vi "m100ProgramCheck.vi"() -> ()   [LabVIEW 2012]
uses:
  <vilib>/addons/database/Auxilliary.llb/DB Tools Cursor Type.ctl
  <vilib>/addons/database/Connection.llb/DB Tools Open Connec (Path).vi
  <vilib>/addons/database/Connection.llb/Conn Execute.vi
  <vilib>/addons/database/Recordset.llb/Rec Fetch Recordset Data (R).vi
  <vilib>/addons/database/Recordset.llb/Rec Destroy - Connection.vi
  <vilib>/addons/database/Recordset.llb/Rec Fetch String Data (R).vi
  <vilib>/addons/database/Recordset.llb/Rec Fetch Integer Data (R).vi
  <vilib>/addons/database/_DB Variant To Data/Database Variant To Data.xnode
  <vilib>/addons/database/NI_Database_API.lvlib
  <vilib>/Utility/SMTP/NI_SMTPEmail.lvlib
panel:
  out "x = y?":bool
  out "data":i32
  out "array":string[][](array[string])
  out "concatenated string 2":string
  out "concatenated string":string
  out "data 5":string
  out "error out":errorcluster
  out "recordset data":variant[][](array[variant])
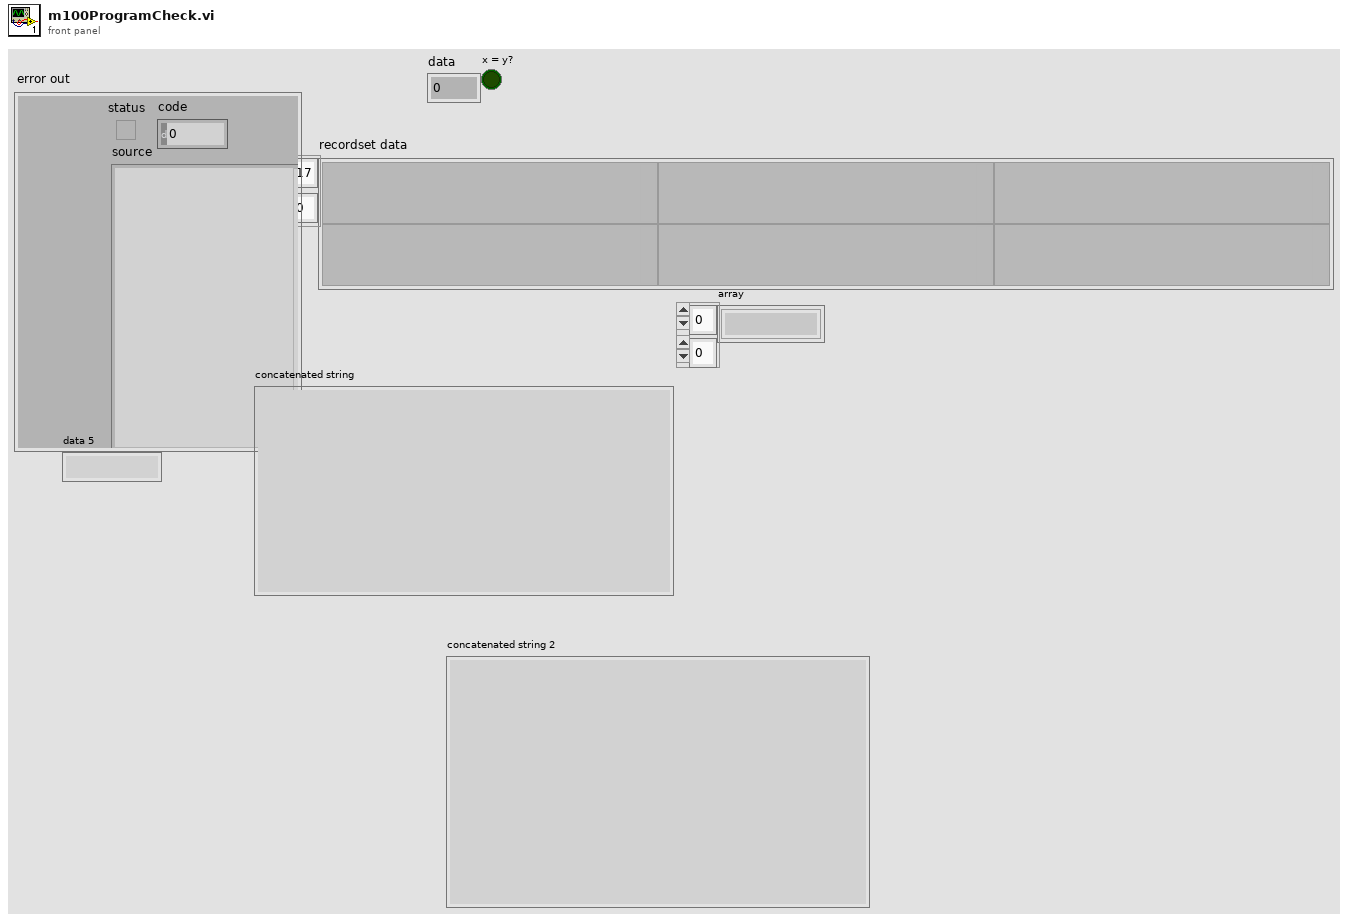
[diagram p1: front panel]
types:
  T1 = typedef "NI_Database_API.lvlib/DB Tools Cursor Type.ctl" = enum16{"forward-only", "keyset", "dynamic", "static"}
  T2 = typedef "NI_Database_API.lvlib/Conn ObjectReference.ctl" = refnum<k1>
  T3 = typedef "NI_Database_API.lvlib/Rec ObjectReference.ctl" = refnum<k1>
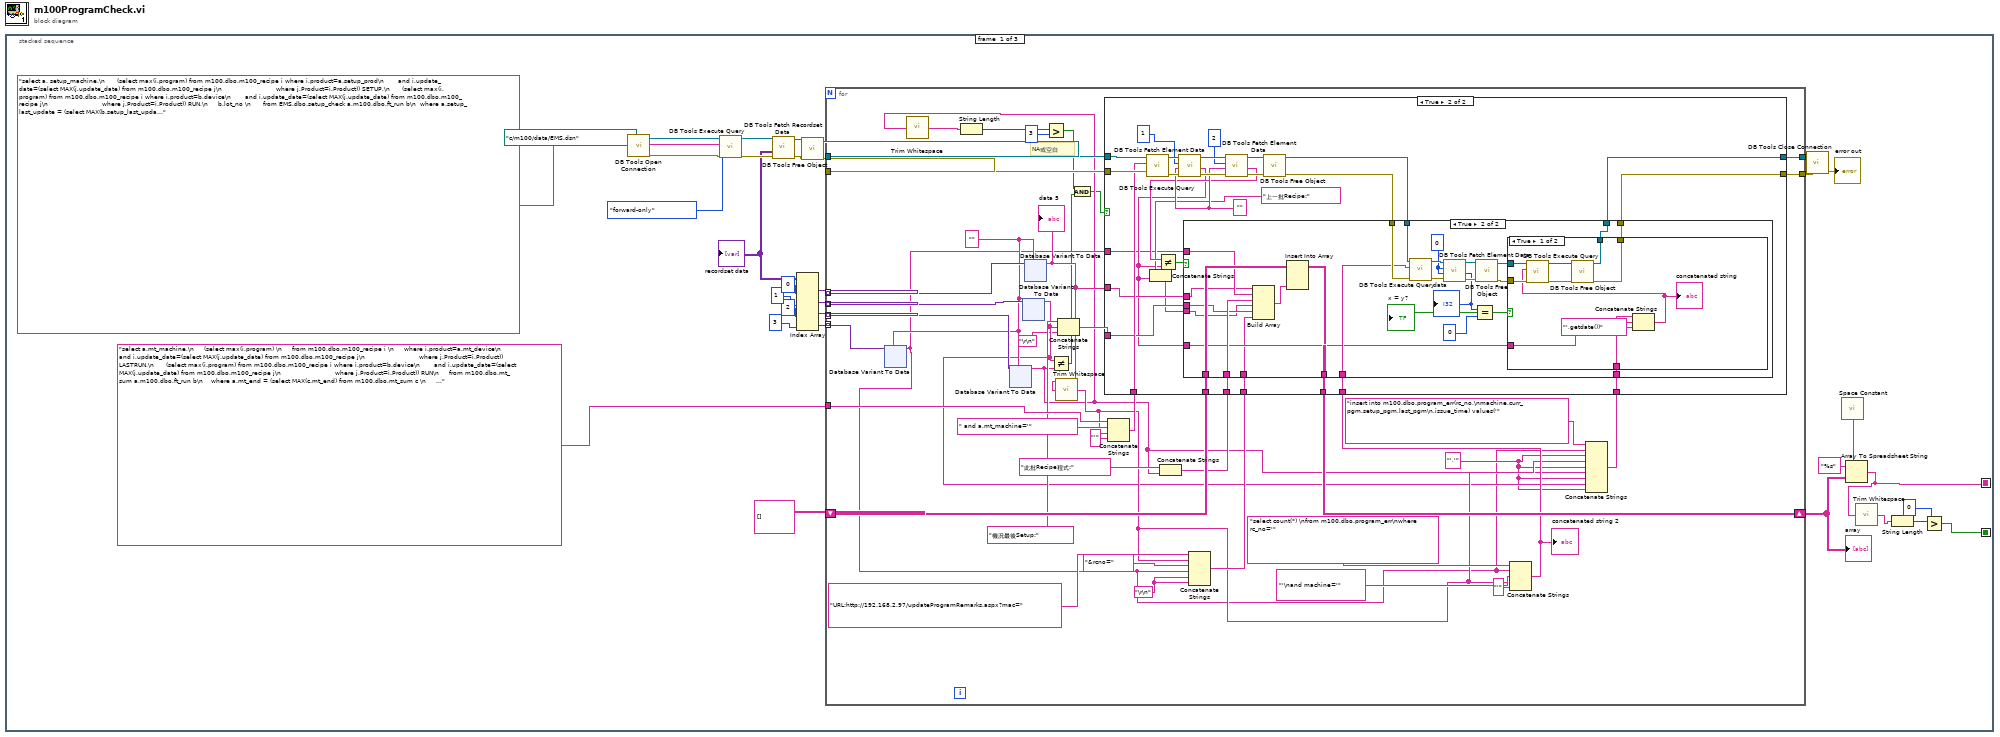
[diagram p0: block diagram]
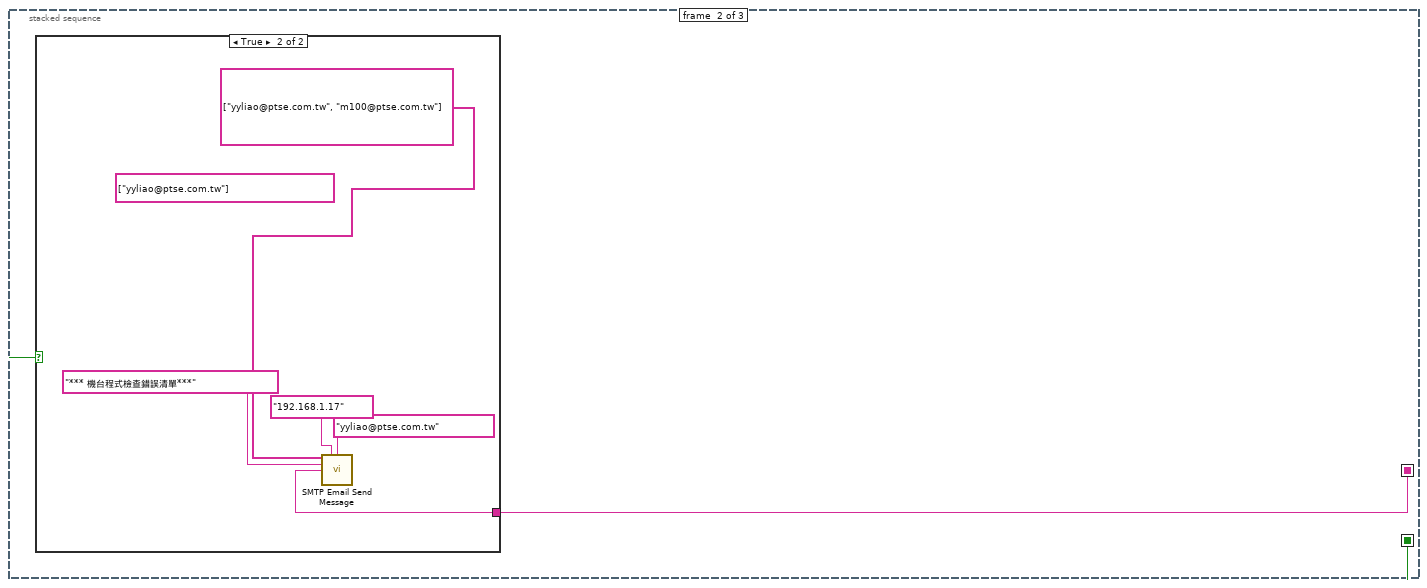
[diagram p5: hidden frame]
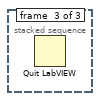
[diagram p7: hidden frame]
diagram:
  n1 = stacked-sequence {
    seq-local: [w5 _ _] -> [_ w279 _]
    seq-local: [w1 _ _] -> [_ w278 _]
    frame #0 {
      n2 = call-poly <vilib>:"DB Tools Open Connection.vi"("connection information"=path "c:/m100/data/EMS.dsn") -> ("error out"=w12:errorcluster, "connection reference"=w13:T2)  [unwired: 7 in]
      n3 = call-poly <vilib>:"DB Tools Execute Query.vi"("error in (no error)"=w12, "cursor type"=DB_Tools_Cursor_Type."forward-only", "SQL query"="select a. setup_machine,\n      (select max(i.program) from m100.dbo.m100_recipe i where i.product=a.setup_prod\n       and i.update_date=(select MAX(j.update_date) from m100.dbo.m100_recipe j\n                           where j.Product=i.Product)) SETUP,\n      (select max(i.program) from m100.dbo.m100_recipe i where i.product=b.device\n       and i.update_date=(select MAX(j.update_date) from m100.dbo.m100_recipe j\n                           where j.Product=i.Product)) RUN,\n     b.lot_no \n      from EMS.dbo.setup_check a,m100.dbo.ft_run b\n  where a.setup_last_update = (select MAX(b.setup_last_update) from EMS.dbo.setup_check b\n                               where b.setup_machine=a.setup_machine)\n    and a.setup_machine=b.machine\n    and b.lot_no like 'A%'\n    and b.station='MT'\n    and b.lot_no not in (select d.rc_no from m100.dbo.program_err d \n                         where d.machine = b.machine\n                           and LEN(d.owner) > 0)\norder by a.setup_machine", "connection reference"=w13) -> ("error out"=w31:errorcluster, "recordset reference"=w32:T3)  [unwired: 4 in]
      n4 = call-poly <vilib>:"DB Tools Fetch Recordset Data.vi"("error in (no error)"=w31, "recordset reference"=w32) -> ("error out"=w29:errorcluster, "recordset data"=w26:variant[][], "recordset reference out"=w30:T3)  [unwired: 3 in]
      "recordset data" <- w26
      n5 = Index Array(array=w26, index (col) #1=0 ("disabled index (col)"), index (col) #2=1 ("index (col)"), index (col) #3=2 ("index (col)"), index (col) #4=3 ("index (col)")) -> (element #1=w22:variant[], element #2=w21:variant[], element #3=w20:variant[], element #4=w6:variant[])  [unwired: 4 in]
      n6 = call-poly <vilib>:"DB Tools Free Object.vi"("error in (no error)"=w29, "recordset reference"=w30) -> ("error out"=w16:errorcluster, "connection reference"=w17:T2)  [unwired: 8 in]
      n7 = for {
        tunnel: w22 -> [w75] mode=indexing
        tunnel: w21 -> [w74] mode=indexing
        tunnel: w20 -> [w73] mode=indexing
        shift-right: [w62] -> w8
        shift-left: string[][] [] ("array") -> [w65]
        tunnel: w17 -> [w72]
        tunnel: w16 -> [w71]
        tunnel: [w70] -> w15
        tunnel: [w69] -> w14
        tunnel: "select a.mt_machine,\n     (select max(i.program) \n     from m100.dbo.m100_recipe i \n     where i.product=a.mt_device\n       and i.update_date=(select MAX(j.update_date) from m100.dbo.m100_recipe j\n                           where j.Product=i.Product)) LASTRUN,\n      (select max(i.program) from m100.dbo.m100_recipe i where i.product=b.device\n       and i.update_date=(select MAX(j.update_date) from m100.dbo.m100_recipe j\n                           where j.Product=i.Product)) RUN\n     from m100.dbo.mt_sum a,m100.dbo.ft_run b\n    where a.mt_end = (select MAX(c.mt_end) from m100.dbo.mt_sum c \n                       where c.mt_machine=a.mt_machine)\n      and a.mt_machine=b.machine\n      and b.station='MT'     " -> [w68]
        tunnel: w6 -> [w56] mode=indexing
        w41 = "\r\n"
        w44 = "','" ("string")
        w55 = ""
        # "NA或空白"
        n8 = xnode "Database Variant To Data"("database variant"=w56, "type"=w55) -> ("data"=w43:string)  [unwired: 1 in, 1 out]
        n9 = xnode "Database Variant To Data"("database variant"=w73, "type"=w55) -> ("data"=w40:string)  [unwired: 1 in, 1 out]
        n10 = call <vilib>:"Trim Whitespace.vi"("string"=w40) -> ("trimmed string"=w39:string)  [unwired: 1 in]
        n11 = String Length(string=w39) -> (length=w38:i32)
        n12 = xnode "Database Variant To Data"("database variant"=w74, "type"=w55) -> ("data"=w46:string)  [unwired: 1 in, 1 out]
        n13 = xnode "Database Variant To Data"("database variant"=w75, "type"=w55) -> ("data"=w63:string)  [unwired: 1 in, 1 out]
        "data 5" <- w63
        n14 = Greater?(x=w38, y=3) -> (0:w36:bool)
        n15 = Not Equal?(x=w46, y=w40) -> (x != y?=w35:bool)
        n16 = call <vilib>:"Trim Whitespace.vi"("string"=w63) -> ("trimmed string"=w47:string)  [unwired: 1 in]
        n17 = Concatenate Strings("機況最後Setup:" ("string"), w46, "\r\n") -> (w58:string)
        n18 = And(x=w36, y=w35) -> (x .and. y?=w34:bool)
        n19 = Concatenate Strings(w68, " and a.mt_machine='" ("string"), w47, "'" ("string")) -> (w66:string)
        n20 = Concatenate Strings("此批Recipe程式:" ("string"), w40) -> (w60:string)
        n21 = Concatenate Strings("URL:http://192.168.2.97/updateProgramRemarks.aspx?mac=" ("string"), w47, "&rcno=" ("string"), w43, w41, w41) -> (w57:string)
        n22 = Concatenate Strings("select count(*) \nfrom m100.dbo.program_err\nwhere rc_no='" ("string"), w43, "'\nand machine='" ("string"), w47, "'" ("string")) -> (w49:string)
        "concatenated string 2" <- w49
        n23 = Concatenate Strings("insert into m100.dbo.program_err(rc_no,\nmachine,curr_pgm,setup_pgm,last_pgm\n,issue_time) values('" ("string"), w43, w44, w47, w44, w40, w44, w46, w44) -> (w45:string)
        n24 = case shown="True" w34 {
          tunnel: w72 -> [w109 w140]
          tunnel: w71 -> [w108 w139]
          tunnel: [w109 w116] -> w70
          tunnel: [w108 w115] -> w69
          tunnel: w66 -> [_ w136]
          tunnel: w65 -> [w110 w126]
          tunnel: [w110 w125] -> w62
          tunnel: w63 -> [_ w124]
          tunnel: w60 -> [_ w123]
          tunnel: w58 -> [_ w122]
          tunnel: w57 -> [_ w119]
          tunnel: w49 -> [_ w114]
          tunnel: w45 -> [_ w113]
          tunnel: w43 -> [_ w111]
          frame False {
          }
          frame True {
            w132 = ""
            n25 = call-poly <vilib>:"DB Tools Execute Query.vi"("error in (no error)"=w139, "SQL query"=w136, "connection reference"=w140) -> ("error out"=w137:errorcluster, "recordset reference"=w138:T3)  [unwired: 5 in]
            n26 = call-poly <vilib>:"DB Tools Fetch Element Data.vi"("error in (no error)"=w137, "type"=w132, "column index"=1, "recordset reference"=w138) -> ("error out"=w134:errorcluster, "data"=w112:string, "recordset reference out"=w130:T3)  [unwired: 3 in]
            n27 = Concatenate Strings("上一批Recipe:" ("string"), w112) -> (w120:string)
            n28 = call-poly <vilib>:"DB Tools Fetch Element Data.vi"("error in (no error)"=w134, "type"=w132, "column index"=2, "recordset reference"=w130) -> ("error out"=w133:errorcluster, "data"=w128:string, "recordset reference out"=w135:T3)  [unwired: 3 in]
            n29 = Not Equal?(x=w128, y=w112) -> (x != y?=w127:bool)
            n30 = call-poly <vilib>:"DB Tools Free Object.vi"("error in (no error)"=w133, "recordset reference"=w135) -> ("error out"=w117:errorcluster, "connection reference"=w118:T2)  [unwired: 8 in]
            n31 = case shown="True" w127 {
              tunnel: w126 -> [w143 w169]
              tunnel: [w143 w168] -> w125
              tunnel: w124 -> [_ w144]
              tunnel: w123 -> [_ w166]
              tunnel: w122 -> [_ w165]
              tunnel: w120 -> [_ w164]
              tunnel: w119 -> [_ w145]
              tunnel: w118 -> [w142 w163]
              tunnel: w117 -> [w141 w162]
              tunnel: [w142 w150] -> w116
              tunnel: [w141 w149] -> w115
              tunnel: w114 -> [_ w161]
              tunnel: w113 -> [_ w148]
              tunnel: w112 -> [_ w147]
              tunnel: w111 -> [_ w146]
              frame False {
              }
              frame True {
                w156 = 0
                n32 = Build Array(w144, w146, w166, w164, w165, w145) -> (w167:string[])
                n33 = Insert Into Array(array=w169, new element=w167) -> (w168:string[][])  [unwired: 2 in]
                n34 = call-poly <vilib>:"DB Tools Execute Query.vi"("error in (no error)"=w162, "SQL query"=w161, "connection reference"=w163) -> ("error out"=w159:errorcluster, "recordset reference"=w160:T3)  [unwired: 5 in]
                n35 = call-poly <vilib>:"DB Tools Fetch Element Data.vi"("error in (no error)"=w159, "type"=w156, "column index"=w156, "recordset reference"=w160) -> ("error out"=w157:errorcluster, "data"=w155:i32, "recordset reference out"=w158:T3)  [unwired: 3 in]
                "data" <- w155
                n36 = Equal?(x=w155, y=0) -> (x = y?=w153:bool)
                "x = y?" <- w153
                n37 = call-poly <vilib>:"DB Tools Free Object.vi"("error in (no error)"=w157, "recordset reference"=w158) -> ("error out"=w151:errorcluster, "connection reference"=w152:T2)  [unwired: 8 in]
                n38 = case shown="True" w153 {
                  tunnel: w152 -> [w179 w181]
                  tunnel: w151 -> [w178 w180]
                  tunnel: [w175 w181] -> w150
                  tunnel: [w174 w180] -> w149
                  tunnel: w148 -> [w173 _]
                  tunnel: w147 -> [w172 _]
                  frame True {
                    n39 = Concatenate Strings(w173, w172, "',getdate())" ("string")) -> (w170:string)
                    "concatenated string" <- w170
                    n40 = call-poly <vilib>:"DB Tools Execute Query.vi"("error in (no error)"=w178, "SQL query"=w170, "connection reference"=w179) -> ("error out"=w176:errorcluster, "recordset reference"=w177:T3)  [unwired: 5 in]
                    n41 = call-poly <vilib>:"DB Tools Free Object.vi"("error in (no error)"=w176, "recordset reference"=w177) -> ("error out"=w174:errorcluster, "connection reference"=w175:T2)  [unwired: 8 in]
                  }
                  frame False {
                  }
                }
              }
            }
          }
        }
      }
      "array" <- w8
      n42 = call <vilib>:"DB Tools Close Connection.vi"("error in (no error)"=w14, "connection reference"=w15) -> ("error out"=→"error out":errorcluster)  [unwired: 5 in]
      n43 = call <vilib>:"Space Constant.vi"() -> ("String"=w18:string)
      n44 = Array To Spreadsheet String(delimiter (Tab)=w18, array=w8, 3:"%s" ("format string")) -> (spreadsheet string=w5:string)
      n45 = call <vilib>:"Trim Whitespace.vi"("string"=w5) -> ("trimmed string"=w4:string)  [unwired: 1 in]
      n46 = String Length(string=w4) -> (length=w3:i32)
      n47 = Greater?(x=w3, y=0) -> (0:w1:bool)
    }
    frame #1 {
      n48 = case shown="True" w278 {
        tunnel: w279 -> [_ w281]
        frame False {
        }
        frame True {
          (unwired) string[] ["yyliao@ptse.com.tw"] ("recipients")
          n49 = call <vilib>:"SMTP Email Send Message.vi"("recipients"=string[] ["yyliao@ptse.com.tw", "m100@ptse.com.tw"], "mail server"="192.168.1.17", "return address"="yyliao@ptse.com.tw", "subject ([No Subject])"="*** 機台程式檢查錯誤清單***", "message"=w281) -> ()  [unwired: 9 in, 2 out]
        }
      }
    }
    frame #2 {
      n50 = Quit LabVIEW() -> ()  [unwired: 1 in]
    }
  }
